vi "parse_header.vi"   [LabVIEW 2015, in "lv-dropbox.lvlib"]
uses:
  lv-dropbox.lvlib
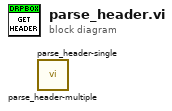
[diagram p0: block diagram]
diagram:
  n1 = call "parse_header-multiple.vi"() -> ()  [unwired: 10 in, 2 out]
  n2 = call "parse_header-single.vi"() -> ()  [unwired: 10 in, 2 out]
